vi "globalSetUp.vi"(8 "error in":errorcluster, 11 "testcase-CSMChainMode in":refnum<class "testcase-CSMChainMode.lvclass">) -> (0 "error out":errorcluster, 3 "testcase-CSMChainMode out":refnum<class "testcase-CSMChainMode.lvclass">)   [LabVIEW 2017, in "testcase-CSMChainMode.lvclass"]
uses:
  testcase-CSMChainMode.lvclass
  <vilib>/addons/_JKI Toolkits/VI Tester/TestCase.llb/TestCase.lvclass
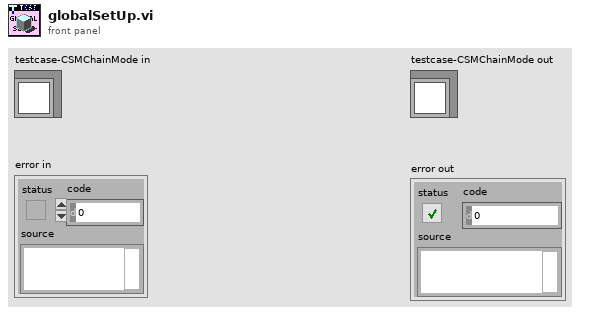
[diagram p1: front panel]
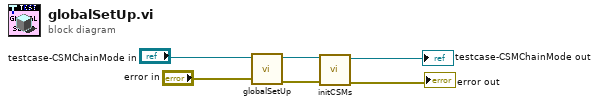
[diagram p0: block diagram]
diagram:
  n1 = call-parent "globalSetUp.vi"("error in (no error)"="error in", "TestCase in"="testcase-CSMChainMode in") -> ("error out"=w1:errorcluster, "TestCase out"=w3:refnum<class "testcase-CSMChainMode.lvclass">)  [unwired: 8 in]
  n2 = call "initCSMs.vi"("error in (no error)"=w1, "TestCase in"=w3) -> ("error out"=→"error out":errorcluster, "TestCase out"=→"testcase-CSMChainMode out":refnum<class "testcase-CSMChainMode.lvclass">)  [unwired: 8 in]
